vi "ReadUarmCoordinatesEDIT.vi"() -> ()   [LabVIEW 2018]
doc: "Example interface for controlling uArm Swift Pro."
panel:
  in  "Stop Button":bool
  out "match + rest of string":string
  out "substring before match":string
  in  "G Code Command":string="#n\\sP2220\\n\\s"
  in  "Write Buffer":string="G90 G0 X1\n"
  out "read buffer":string="echo:Unknown command: \"sP2220nsððððððððG90sG0sX1n#n P2201\"\n"
  # "G90\\sG0\\sX1\\n"
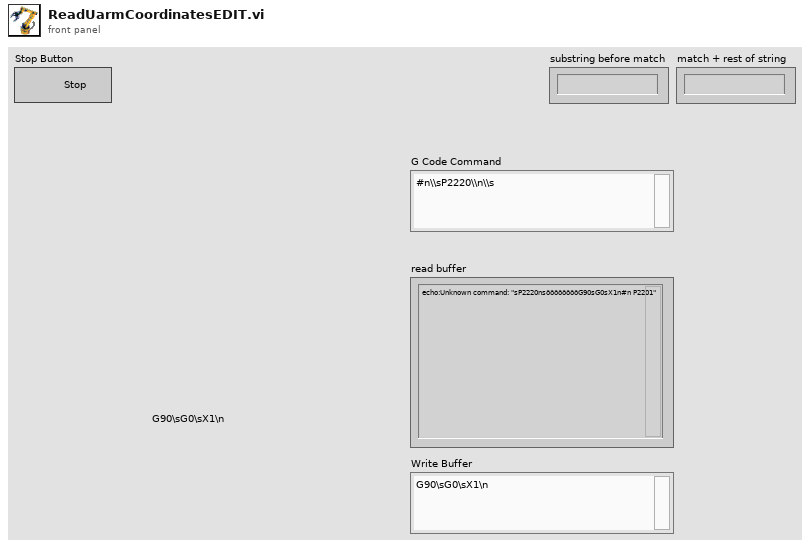
[diagram p1: front panel]
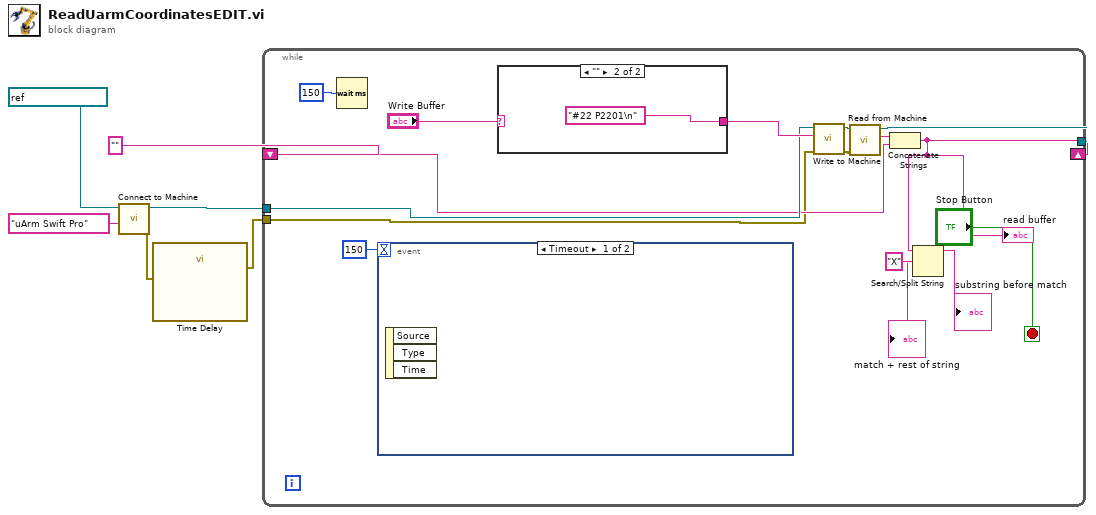
[diagram p0: block diagram]
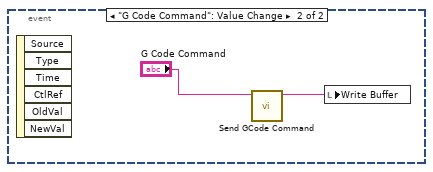
[diagram p2: hidden frame]
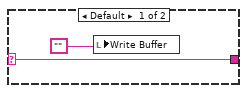
[diagram p3: hidden frame]
diagram:
  n1 = call "Connect to Machine .vi"("Firmware"="uArm Swift Pro", "Machine In"=refnum<visa-resource-name> "ASRL2::INSTR") -> ("error out"=w3:errorcluster, "Machine Out"=w6:refnum<visa-resource-name>)  [unwired: 7 in, 1 out]
  n2 = call "Time Delay"("error in (no error)"=w3) -> ("error out"=w4:errorcluster)  [unwired: 10 in]
  n3 = while {
    tunnel: w6 -> [w16]
    tunnel: w4 -> [w13]
    shift-right: [w11] -> _
    shift-left: "" -> [w15]
    tunnel: [w18] -> _
    stop <- "Stop Button" stop-if-true
    n4 = Wait (ms)(milliseconds to wait=u32 150) -> ()  [unwired: 1 out]
    n5 = event shown="[0] Timeout" {
      selector: _ -> [_ _]
      dyn-events: _ -> [_ _]
      timeout: 150 -> [_ _]
      event Timeout {
        n6 = event-data() -> ()  [unwired: 1 in, 3 out]
      }
      event "G Code Command": Value Change {
        n7 = event-data() -> ()  [unwired: 1 in, 6 out]
        n8 = call "Send GCode Command.vi"("G-Code Command in"="G Code Command") -> ("G-Code Command out"=w24:string)  [unwired: 10 in]
        n9 = local write "Write Buffer"(w24) -> ()
      }
    }
    n10 = case shown="\"\"" "Write Buffer" {
      selector: "Write Buffer" -> [w26 _]
      tunnel: [w26 "#22 P2201\n"] -> w21
      frame Default {
        n11 = local write "Write Buffer"("") -> ()
      }
      frame "" {
      }
    }
    n12 = call "Write to Machine .vi"("error in (no error)"=w13, "G-Code String In"=w21, "Machine In"=w16) -> ("error out"=w19:errorcluster, "Machine Out"=w20:refnum<visa-resource-name>)  [unwired: 7 in]
    n13 = call "Read from Machine.vi"("error in (no error)"=w19, "Machine In"=w20) -> ("read buffer"=w14:string, "Machine Out"=w18:refnum<visa-resource-name>)  [unwired: 7 in, 1 out]
    n14 = Concatenate Strings(w14, w15) -> (w11:string)
    "read buffer" <- w11
    n15 = Search/Split String(string=w11, search string/char (-)="X") -> (substring before match=→"substring before match":string, match + rest of string=→"match + rest of string":string)  [unwired: 1 in, 1 out]
  }
